vi "Finish.vi"   [LabVIEW 2013]
doc: "This VI is called just before exiting. It is expected to close I/O refnum, save collected data, etc."
uses:
  <vilib>/Rock Robotics/WPI/RobotDrive/WPI_RobotDriveGetSetRefNum.vi
  <vilib>/Rock Robotics/WPI/Joystick/WPI_JoystickGetSetRefNum.vi
types:
  T1 = typedef "WPI_GyroDevRef.ctl" = cluster{"DevStatus":errorcluster, "Analog Module":T2, "Analog Channel":T3, "Offset":dbl, "Gain (VoltsPerDegree/Second)":dbl}
  T2 = typedef "FPGA_TypedefAnalogModule.ctl" = enum16{"Analog Module 1", "Analog Module 2"}
  T3 = typedef "FPGA_AIChannel.ctl" = enum8{"AI 1", "AI 2", "AI 3", "AI 4", "AI 5", "AI 6", "AI 7", "AI 8", "Invalid"}
  T4 = typedef "WPI_JoystickDevRef.ctl" = cluster{"Device":T5}
  T5 = typedef "WPI_JoystickDeviceEnum.ctl" = enum16{"USB 1", "USB 2", "USB 3", "USB 4", "Kinect 1", "Kinect 2"}
  T6 = typedef "WPI_RobotDriveDevRef.ctl" = cluster{"DevStatus":errorcluster, "Motors[]":T7[], "Square Inputs":bool, "Max Output":dbl, "Isochronous":bool}
  T7 = typedef "WPI_MotorControlDeviceRef.ctl" = cluster{"DeviceStatus":errorcluster, "Type":enum16{"PWM", "CAN"}, "PWM":cluster{"Digital Module":T8, "PWM Channel":T9, "DeadBand":T10}, "CAN":cluster{"Device Number":u8, "Control Mode":T11, "Semaphore":T12, "Max Vout":dbl}, "Invert":bool, "TransformRef":T13, "InvTransformRef":T13}
  T8 = typedef "FPGA_TypedefDigitalModule.ctl" = enum16{"Digital Module 1", "Digital Module 2"}
  T9 = typedef "FPGA_DIOPWMChannel.ctl" = enum8{"PWM 1", "PWM 2", "PWM 3", "PWM 4", "PWM 5", "PWM 6", "PWM 7", "PWM 8", "PWM 9", "PWM 10", "Invalid"}
  T10 = typedef "WPI_PWMDeadband.ctl" = cluster{"Name":string, "maxPositivePwm":i32, "minPositivePwm":i32, "centerPwm":i32, "maxNegativePwm":i32, "minNegativePwm":i32, "angularRange":u16}
  T11 = typedef "WPI_CANJaguar_ControlMode.ctl" = enum8{"Percent VBus", "Current", "Speed", "Position", "Voltage"}
  T12 = typedef "Semaphore RefNum" = refnum<k1>
  T13 = typedef "WPI_PWMTransform_ConPane.ctl" = refnum<vi>
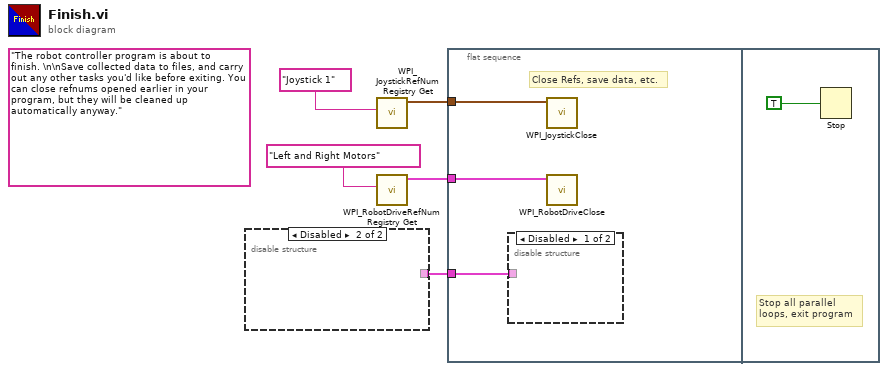
[diagram p0: block diagram]
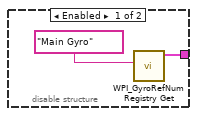
[diagram p2: hidden frame]
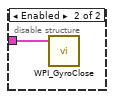
[diagram p3: hidden frame]
diagram:
  (unwired) "The robot controller program is about to finish. \n\nSave collected data to files, and carry out any other tasks you'd like before exiting. You can close refnums opened earlier in your program, but they will be cleaned up automatically anyway."
  n1 = disable-structure shown="Disabled" {
    disable-tunnel: [w6 _] -> w1
    frame Enabled {
      n2 = call <vilib>:"WPI_GyroRefNum Registry Get.vi"("refnum name"="Main Gyro") -> ("GyroDevRef"=w6:T1)  [unwired: 9 in, 1 out]
    }
    frame Disabled {
    }
  }
  n3 = call <vilib>:"WPI_JoystickRefNum Registry Get.vi"("refnum name"="Joystick 1") -> ("JoystickDevRef"=w2:T4)  [unwired: 1 in, 9 out]
  n4 = call <vilib>:"WPI_RobotDriveRefNum Registry Get.vi"("refnum name"="Left and Right Motors") -> ("RobotDriveDevRef"=w3:T6)  [unwired: 1 in, 9 out]
  n5 = flat-sequence {
    tunnel: w3 -> [w10]
    tunnel: w2 -> [w9]
    tunnel: w1 -> [w8]
    frame #0 {
      # "Close Refs, save data, etc."
      n6 = disable-structure shown="Disabled" {
        disable-tunnel: w8 -> [_ w11]
        frame Disabled {
        }
        frame Enabled {
          n7 = call <vilib>:"WPI_GyroClose.vi"("GyroDevRef"=w11) -> ()  [unwired: 1 in, 10 out]
        }
      }
      n8 = call <vilib>:"WPI_JoystickClose.vi"("JoystickDevRef"=w9) -> ()  [unwired: 11 out]
      n9 = call <vilib>:"WPI_RobotDriveClose.vi"("RobotDriveDevRef"=w10) -> ()  [unwired: 1 in, 10 out]
    }
    frame #1 {
      # "Stop all parallel\nloops, exit program"
      n10 = Stop(stop? (T)=TRUE ("Quit")) -> ()
    }
  }
